vi "Open DAQ Configuration.vi"(8 "Error In":errorcluster) -> (0 "Error Out":errorcluster, 2 "DAQ Device Settings":T1={"Analog Input Channel"="Dev1/ai0", "AImin[V]"=0, "AImax[V]"=5, "Analog Output Channel"="Dev1/ao0", "AOmin[V]"=0, "AOmax[V]"=5} {"AOmax[V]" min=-10 max=10 step=1 format="%.0g"; "AOmin[V]" min=-10 max=10 step=1 format="%.0g"; "AImax[V]" min=-10 max=10 step=1 format="%.0g"; "AImin[V]" min=-10 max=10 step=1 format="%.0g"})   [LabVIEW 2018]
uses:
  <vilib>/Utility/config.llb/Read Key (String).vi
  <vilib>/Utility/config.llb/Read Key (I32).vi
  <vilib>/Utility/config.llb/NI_LVConfig.lvlib
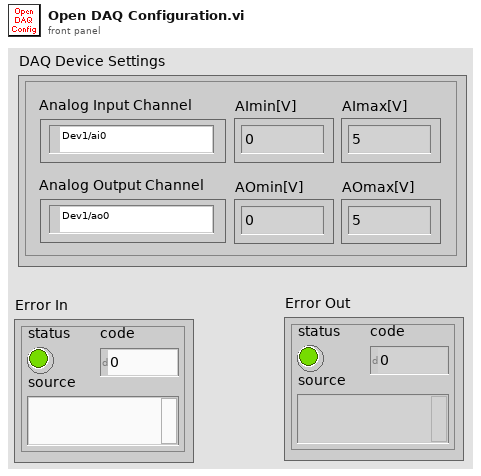
[diagram p1: front panel]
types:
  T1 = cluster{"Analog Input Channel":tag, "AImin[V]":i32, "AImax[V]":i32, "Analog Output Channel":tag, "AOmin[V]":i32, "AOmax[V]":i32}
  T2 = typedef "NI_LVConfig.lvlib/Config Data RefNum.ctl" = refnum<k1>
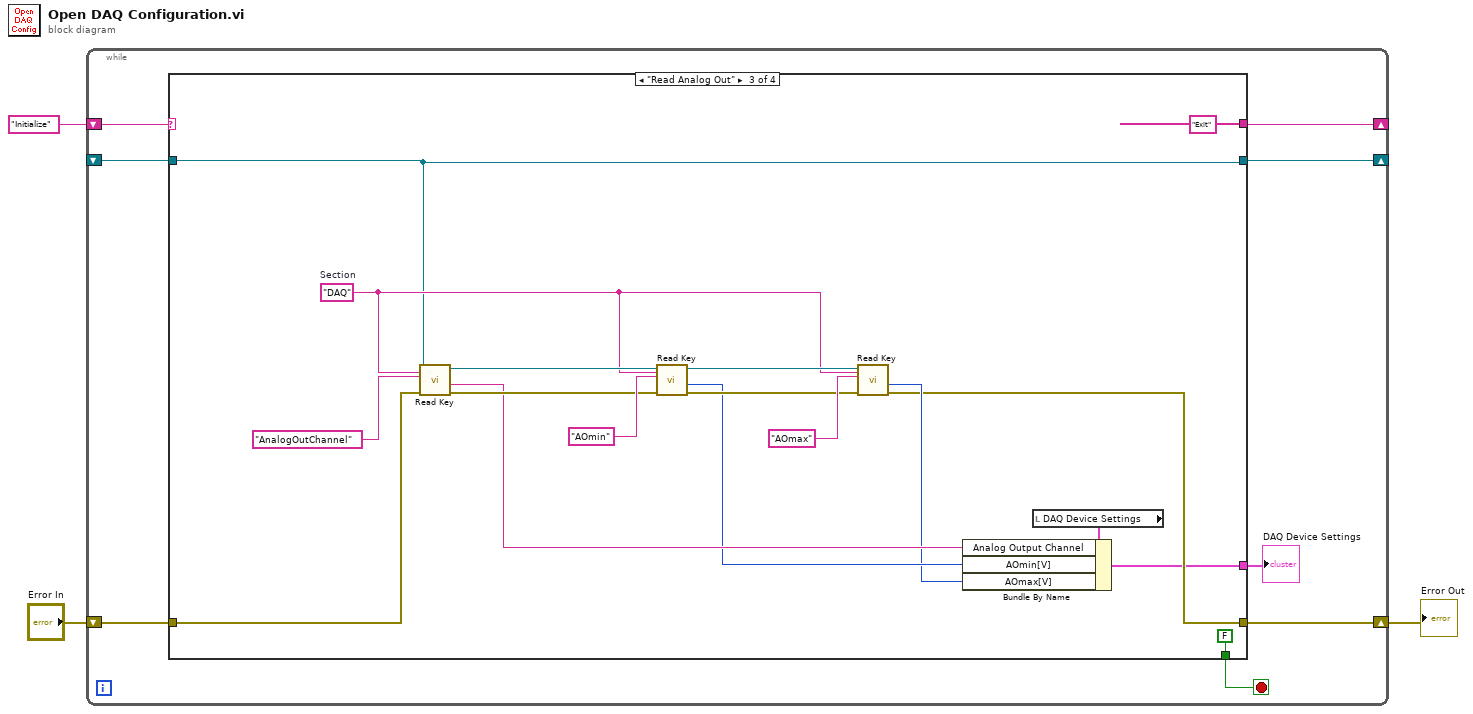
[diagram p0: block diagram]
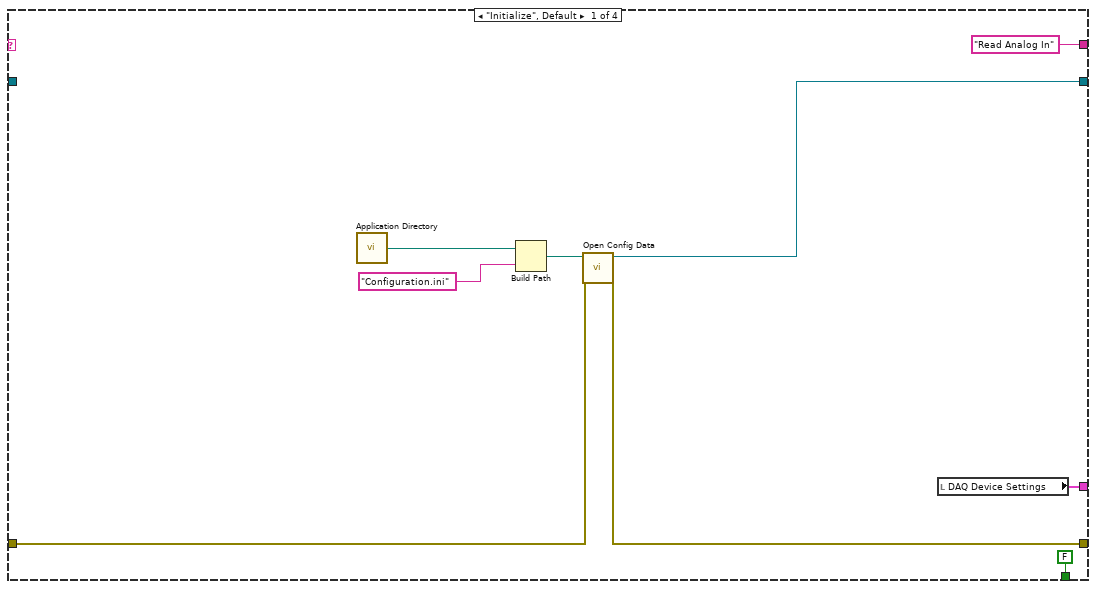
[diagram p2: hidden frame]
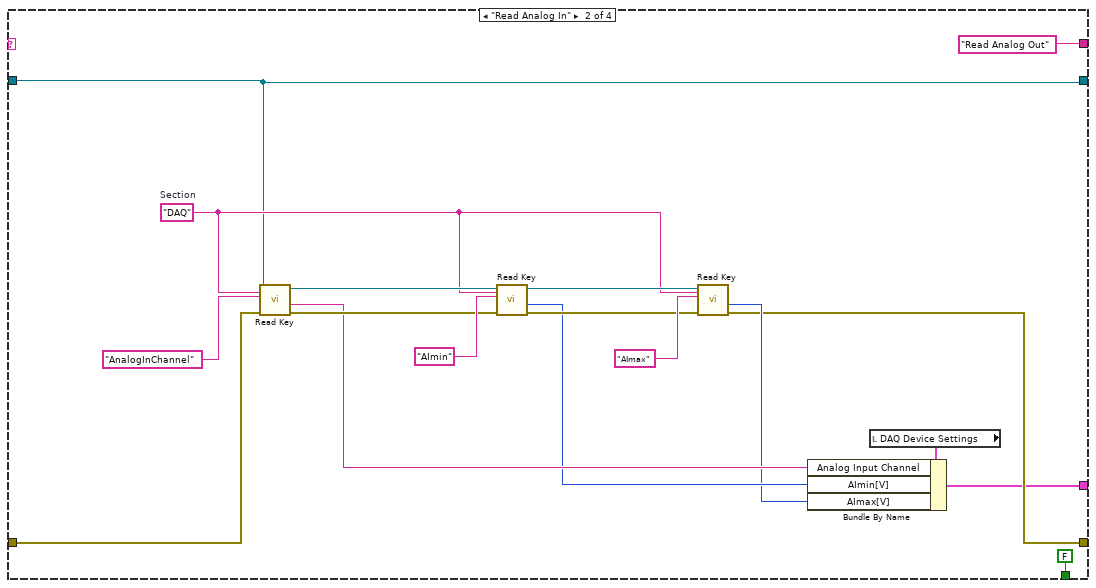
[diagram p3: hidden frame]
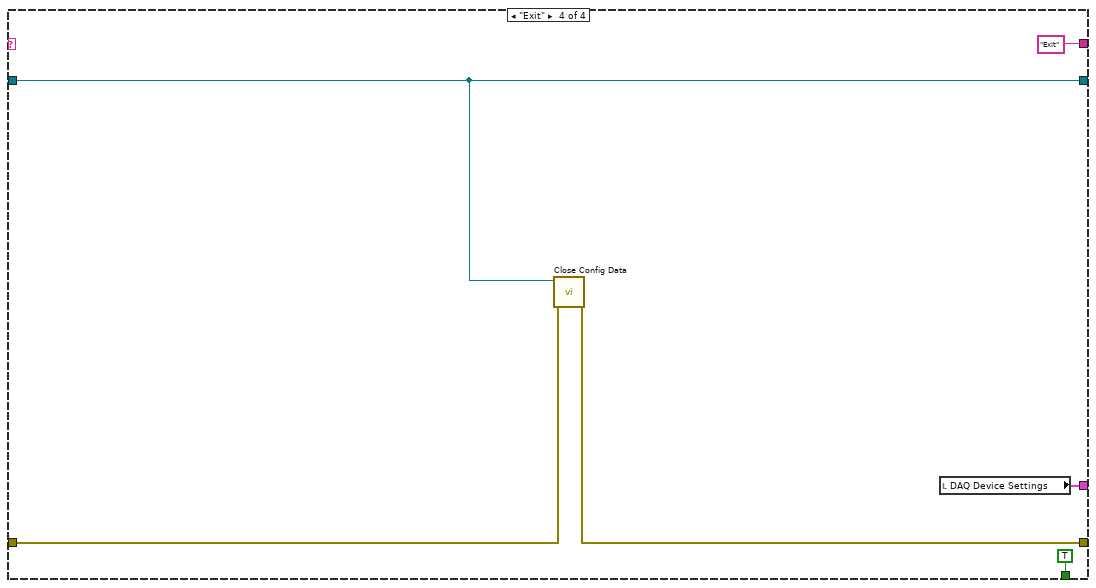
[diagram p4: hidden frame]
diagram:
  n1 = while {
    shift-right: [w7] -> _
    shift-left: "Initialize" ("key") -> [w11]
    shift-right: [w8] -> _
    shift-left: _ -> [w10]
    shift-right: [w5] -> w1
    shift-left: "Error In" -> [w9]
    stop <- w6 stop-if-true
    n2 = case shown="\"Read Analog Out\"" w11 {
      tunnel: w10 -> [_ w23 w41 w60]
      tunnel: w9 -> [w14 w28 w46 w59]
      tunnel: [w15 w23 w41 w60] -> w8
      tunnel: ["Read Analog In" ("key") "Read Analog Out" ("key") "Exit" ("key") "Exit" ("key")] -> w7
      tunnel: [FALSE FALSE FALSE TRUE] -> w6
      tunnel: [w13 w24 w42 w58] -> w5
      tunnel: [w12 w21 w39 w57] -> w4
      frame "Initialize", Default {
        n3 = call <vilib>:"Application Directory.vi"() -> ("Application Directory"=w18:path)
        n4 = Build Path(base path=w18, name or relative path="Configuration.ini") -> (appended path=w16:path)
        n5 = call <vilib>:"Open Config Data.vi"("error in (no error)"=w14, "configuration file path"=w16) -> ("error out"=w13:errorcluster, "refnum"=w15:T2)  [unwired: 7 in, 1 out]
        n6 = local read "DAQ Device Settings"() -> (w12:T1)
      }
      frame "Read Analog In" {
        w29 = "DAQ"  # Section
        n7 = call-poly <vilib>:"Read Key.vi"("section"=w29, "error in (no error)"=w28, "key"="AnalogInChannel", "refnum"=w23) -> ("error out"=w35:errorcluster, "value"=w27:string, "refnum out"=w34:T2)  [unwired: 4 in, 1 out]
        n8 = call-poly <vilib>:"Read Key.vi"("section"=w29, "error in (no error)"=w35, "key"="AImin", "refnum"=w34) -> ("error out"=w30:errorcluster, "value"=w26:i32, "refnum out"=w31:T2)  [unwired: 4 in, 1 out]
        n9 = call-poly <vilib>:"Read Key.vi"("section"=w29, "error in (no error)"=w30, "key"="AImax", "refnum"=w31) -> ("error out"=w24:errorcluster, "value"=w25:i32)  [unwired: 4 in, 2 out]
        n10 = local read "DAQ Device Settings"() -> (w22:T1)
        n11 = Bundle By Name(cluster=w22, "Analog Input Channel"=w27, "AImin[V]"=w26, "AImax[V]"=w25) -> (w21:T1)
      }
      frame "Read Analog Out" {
        w47 = "DAQ"  # Section
        n12 = call-poly <vilib>:"Read Key.vi"("section"=w47, "error in (no error)"=w46, "key"="AnalogOutChannel", "refnum"=w41) -> ("error out"=w53:errorcluster, "value"=w45:string, "refnum out"=w52:T2)  [unwired: 4 in, 1 out]
        n13 = call-poly <vilib>:"Read Key.vi"("section"=w47, "error in (no error)"=w53, "key"="AOmin", "refnum"=w52) -> ("error out"=w48:errorcluster, "value"=w44:i32, "refnum out"=w49:T2)  [unwired: 4 in, 1 out]
        n14 = call-poly <vilib>:"Read Key.vi"("section"=w47, "error in (no error)"=w48, "key"="AOmax", "refnum"=w49) -> ("error out"=w42:errorcluster, "value"=w43:i32)  [unwired: 4 in, 2 out]
        n15 = local read "DAQ Device Settings"() -> (w40:T1)
        n16 = Bundle By Name(cluster=w40, "Analog Output Channel"=w45, "AOmin[V]"=w44, "AOmax[V]"=w43) -> (w39:T1)
      }
      frame "Exit" {
        n17 = call <vilib>:"Close Config Data.vi"("error in (no error)"=w59, "refnum"=w60) -> ("error out"=w58:errorcluster)  [unwired: 8 in, 1 out]
        n18 = local read "DAQ Device Settings"() -> (w57:T1)
      }
    }
    "DAQ Device Settings" <- w4
  }
  "Error Out" <- w1
